vi "Manual Control.vi"(6 "Wrist Setpoint":dbl, 7 "Description":string, 8 "Command Info In":T1, 9 "Elbow Setpoint":dbl, 10 "Shoulder Setpoint":dbl, 11 "Turret Setpoint":dbl) -> (0 "Command Info Out":T1)   [LabVIEW 2018]
doc: "This template is useful for immediate subsystem actions that do not need deadband filtering\n\nBe sure to right-click and select New from Template and save with a new command name."
uses:
  <vilib>/Rock Robotics/WPI/Framework/Command Status Info.ctl
  <vilib>/Rock Robotics/WPI/Framework/Completion Status.ctl
  <vilib>/Rock Robotics/WPI/Framework/Completion Notifier.ctl
  Implementation/Arm Setpoints.ctl
  Implementation/Arm Operations.ctl
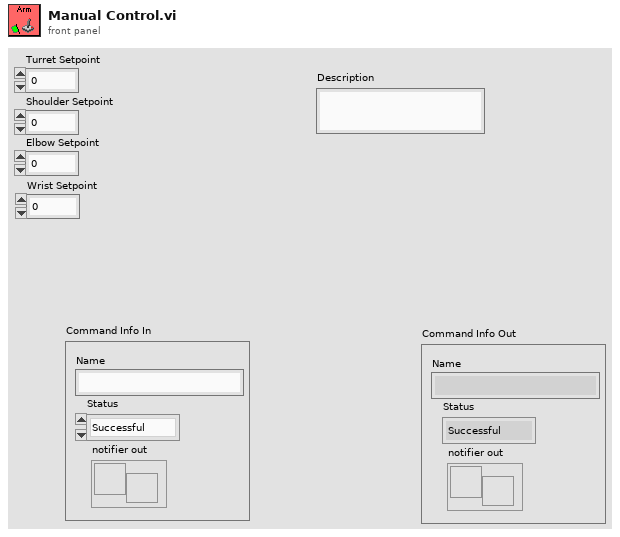
[diagram p1: front panel]
types:
  T1 = typedef "Command Status Info.ctl" = cluster{"Name":string, "Status":T2, "notifier out":T3}
  T2 = typedef "Completion Status.ctl" = enum16{"Successful", "Aborted", "Incomplete"}
  T3 = typedef "Completion Notifier.ctl" = refnum<notifier>
  T4 = typedef "Arm Setpoints.ctl" = cluster{"Operation":T5, "Turret Setpoint":dbl, "Shoulder Setpoint":dbl, "Elbow Setpoint":dbl, "Wrist Setpoint":dbl}
  T5 = typedef "Arm Operations.ctl" = enum16{"Reserve", "Read Current", "Immediate", "Move arm to position"}
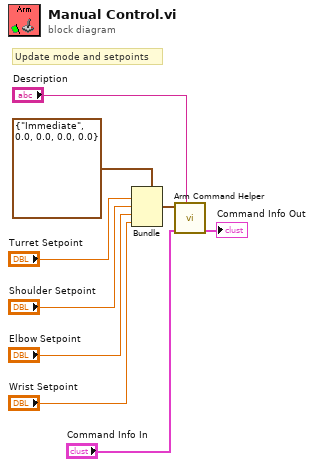
[diagram p0: block diagram]
diagram:
  # "Update mode and setpoints"
  n1 = Bundle(cluster=T4 {"Operation"=enum."Immediate", "Turret Setpoint"=0.0, "Shoulder Setpoint"=0.0, "Elbow Setpoint"=0.0, "Wrist Setpoint"=0.0} ("SubSystem Data"), "Turret Setpoint"="Turret Setpoint", "Shoulder Setpoint"="Shoulder Setpoint", "Elbow Setpoint"="Elbow Setpoint", "Wrist Setpoint"="Wrist Setpoint") -> (w5:T4)  [unwired: 1 in]
  n2 = call "Arm Command Helper.vi"("Description"="Description", "Command Info In"="Command Info In", "SubSystem Data"=w5) -> ("Command Info Out"=→"Command Info Out":T1)  [unwired: 6 in, 2 out]
